vi "findr.vi"(8 "thresh":i32=1, 9 "esize":i32=1, 11 "inp array":i32[][](array[numeric])) -> (3 "locs":i32[][](array[numeric]))   [LabVIEW 2020]
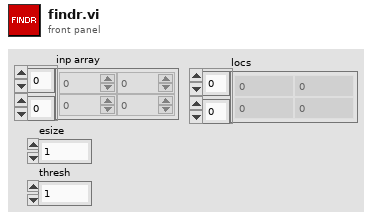
[diagram p1: front panel]
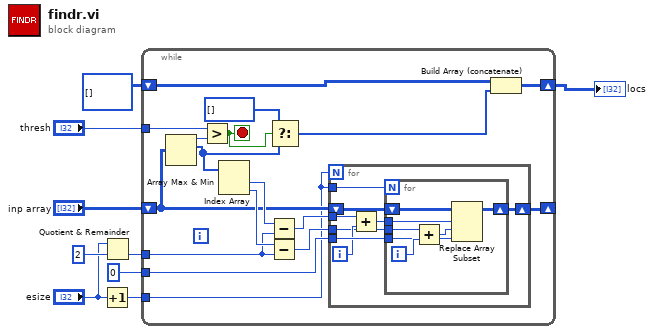
[diagram p0: block diagram]
diagram:
  n1 = Increment(x="esize") -> (x+1=w7:i32)
  n2 = Quotient & Remainder(x="esize", y=2) -> (floor(x/y)=w8:i32)  [unwired: 1 out]
  n3 = while {
    tunnel: "thresh" -> [w26]
    tunnel: w8 -> [w22]
    tunnel: w7 -> [w17]
    tunnel: 0 ("y") -> [w19]
    shift-right: [w16] -> _
    shift-left: "inp array" -> [w21]
    shift-right: [w14] -> w5
    shift-left: i32[][] [] -> [w15]
    stop <- w13 stop-if-true
    n4 = Array Max & Min(array=w21) -> (max value=w25:i32, max index (indices)=w10:i32[])  [unwired: 2 out]
    n5 = Greater?(x=w26, y=w25) -> (0:w13:bool)
    n6 = Index Array(array=w10) -> (element #1=w24:i32, element #2=w23:i32)  [unwired: 2 in]
    n7 = Subtract(x=w24, y=w22) -> (x-y=w18:i32)
    n8 = Subtract(x=w23, y=w22) -> (x-y=w20:i32)
    n9 = Select(t=i32[] [], s=w13, f=w10) -> (s? t:f=w11:i32[])
    n10 = for {
      N: w17 -> [_]
      tunnel: w20 -> [w28]
      tunnel: w19 -> [w33]
      shift-right: [w32] -> w16
      shift-left: w21 -> [w34]
      tunnel: w18 -> [w30]
      tunnel: w17 -> [w27]
      i -> [w31]
      n11 = Add(x=w30, y=w31) -> (x+y=w29:i32)
      n12 = for {
        N: w27 -> [_]
        tunnel: w29 -> [w40]
        tunnel: w28 -> [w37]
        tunnel: w33 -> [w35]
        shift-right: [w39] -> w32
        shift-left: w34 -> [w41]
        i -> [w38]
        n13 = Add(x=w37, y=w38) -> (x+y=w36:i32)
        n14 = Replace Array Subset(array=w41, new element=w35, index (row)=w40, index (col)=w36) -> (w39:i32[][])
      }
    }
    n15 = Build Array (concatenate)(w15, w11) -> (w14:i32[][])
  }
  "locs" <- w5
